vi "Count Actors.vi"(10 "Increment?":bool) -> ()   [LabVIEW 2021, in "AAM.lvlib" / "LVCAM.lvclass"]
uses:
  LVCAM.lvclass
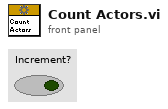
[diagram p1: front panel]
types:
  T1 = enum32{"Invalid", "Standard", "Closed", "Hidden", "Minimized", "Maximized"}
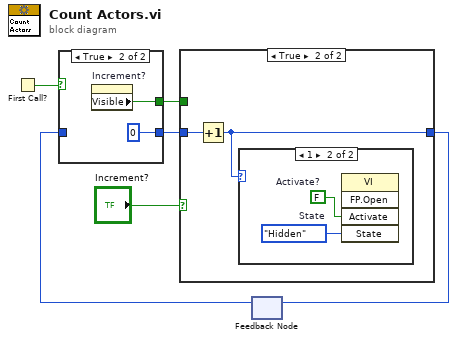
[diagram p0: block diagram]
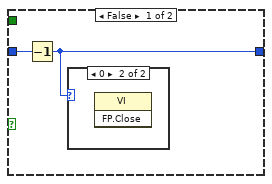
[diagram p2: hidden frame]
diagram:
  n1 = First Call?() -> (First Call?: T/F=w5:bool)
  n2 = feedback #1() -> (w2:u32)  [unwired: 1 in]
  n3 = case shown="True" w5 {
    tunnel: w2 -> [w7 _]
    tunnel: [w7 u32 0] -> w4
    tunnel: [_ w8] -> w1
    frame False {
    }
    frame True {
      n4 = property on="Increment?" class="Bool (strict)"() -> ("Visible"=w8:bool)  [unwired: 2 in, 2 out]
    }
  }
  n5 = case shown="True" "Increment?" {
    tunnel: w4 -> [w11 w13]
    tunnel: [w10 w12] -> w3
    tunnel: w1 -> [_ _]
    frame False {
      n6 = Decrement(x=w11) -> (x-1=w10:u32)
      n7 = case shown="0" w10 {
        frame Default {
        }
        frame 0 {
          n8 = invoke class="VI" method="FP.Close"() -> ()  [unwired: 3 in, 3 out]
        }
      }
    }
    frame True {
      n9 = Increment(x=w13) -> (x+1=w12:u32)
      n10 = case shown="1" w12 {
        frame Default {
        }
        frame 1 {
          w14 = FALSE  # Activate?
          w15 = T1."Hidden"  # State
          n11 = invoke class="VI" method="FP.Open"("Activate"=w14, "State"=w15) -> ()  [unwired: 3 in, 5 out]
        }
      }
    }
  }
  n12 = feedback-in #1(w3) -> ()
